vi "Read Message.vi"(8 "error in (no error)":errorcluster, 9 "timeout":i32, 11 "TCPIP in":refnum<class "TCPIP.lvclass">) -> (0 "error out":errorcluster, 2 "Message":string, 3 "TCPIP out":refnum<class "TCPIP.lvclass">)   [LabVIEW 2018, in "TCPIP.lvclass"]
uses:
  TCPIP.lvclass
  TCPIP.lvclass/TCPIP.ctl
panel:
  out "error out 2":errorcluster
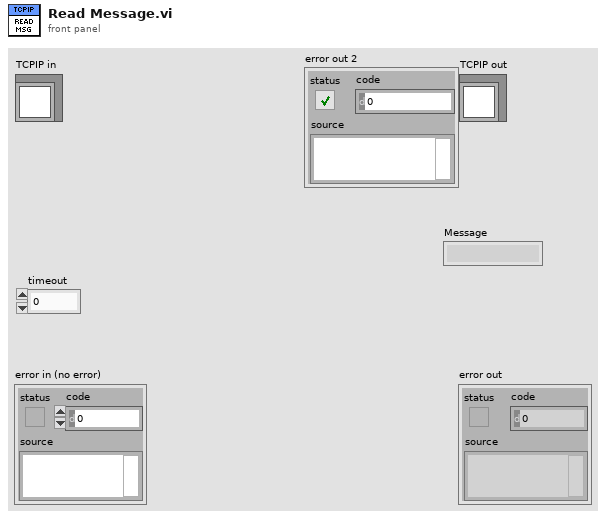
[diagram p1: front panel]
types:
  T1 = enum16{"Standard", "Buffered", "CRLF", "Immediate"}
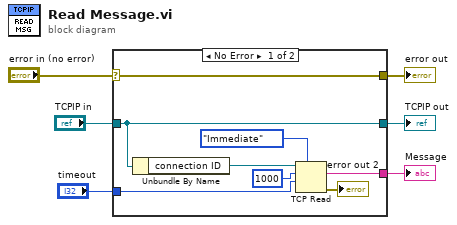
[diagram p0: block diagram]
diagram:
  n1 = case shown="No Error" "error in (no error)" {
    selector: "error in (no error)" -> [w9 w16]
    tunnel: [w9 w16] -> w5
    tunnel: [w14 w15] -> w3
    tunnel: "TCPIP in" -> [w14 w15]
    tunnel: [w12 _] -> w2
    tunnel: "timeout" -> [w11 _]
    frame No Error {
      n2 = Unbundle By Name(w14) -> ("connection ID"=w13:refnum<k5>)
      n3 = TCP Read(connection ID=w13, bytes to read=1000, 7:T1."Immediate" ("mode (standard)"), 9:w11) -> (data out=w12:string, error out=→"error out 2":errorcluster)  [unwired: 1 in, 1 out]
    }
    frame Error {
    }
  }
  "error out" <- w5
  "TCPIP out" <- w3
  "Message" <- w2
